vi "Sentivity Test.vi"() -> ()   [LabVIEW 2018]
uses:
  <vilib>/express/express analysis/Spectral/Block/exnSpectralBlock spectral measurements peak poly.vi
  <vilib>/express/express analysis/Spectral/Block/exnSpectralBlock spectral measurements peak DDT.vi
  <vilib>/express/express analysis/Spectral/XNode/ExpressSpectralMeasurementsBlockNode.xnode
panel:
  out "Avg For 5 Time":dbl
  out "Max @ Peak":dbl[](array[numeric])
  out "Max @ Peak":dbl
  out "Freq Hz":dbl
  in  "Test Senitivity Here":dbl=131.0
  out "FFT 2":dynamicdata(graph)
  out "TD 2":dynamicdata(graph)
  in  "Sample to Read":i32=6400
  in  "Rate":dbl=6400.0
  out "Freq Hz":dbl
  out "Max @ Peak":dbl
  out "FFT":dynamicdata(graph)
  out "TD":dynamicdata(graph)
  in  "stop (F)":bool
  # "校正器使用 394C06\n\n輸出 1g (9.8 m/s^2)\n頻率 159.2 Hz\n\n設定 5 倍取樣量 才能抓到 0.2 Hz"
  # "Senitivity set  1 mV/g in DAQmx"
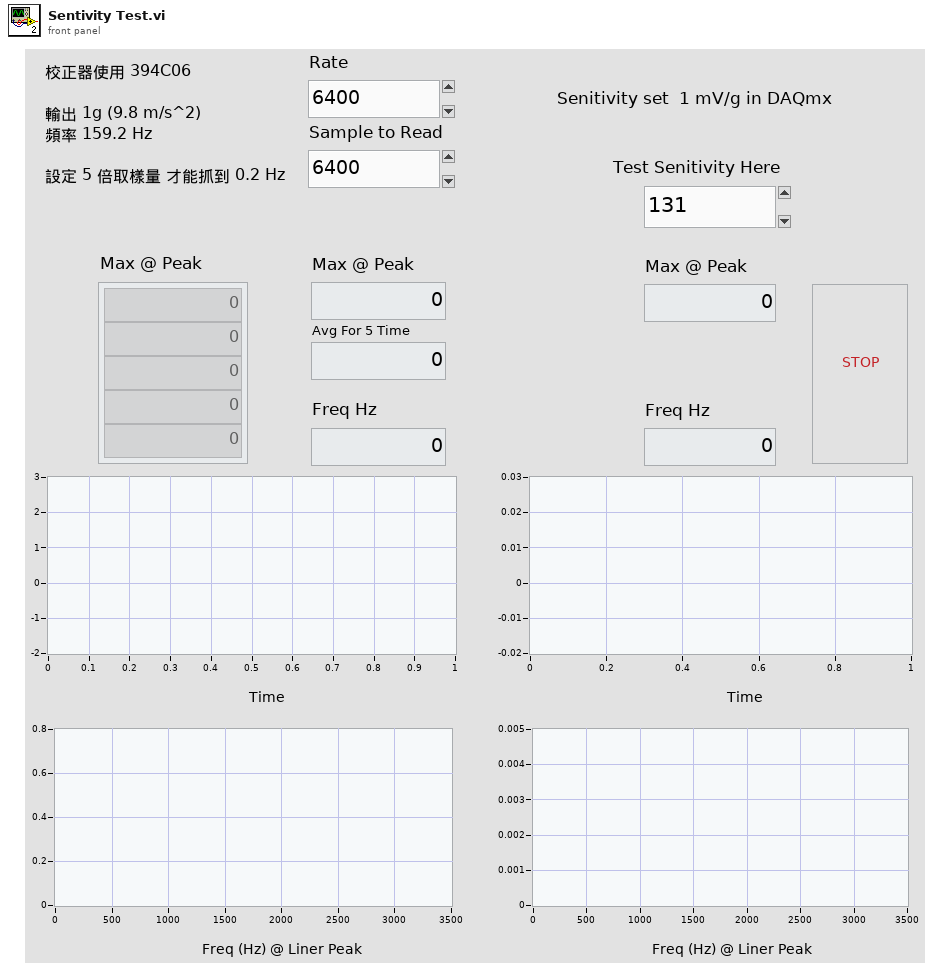
[diagram p1: front panel]
types:
  T1 = cluster{"averaging mode":u16, "weighting mode":u16, "number of averages":u32}
  T2 = cluster{"dB On (F)":bool, "unwrap phase (F)":bool, "convert to degree (F)":bool}
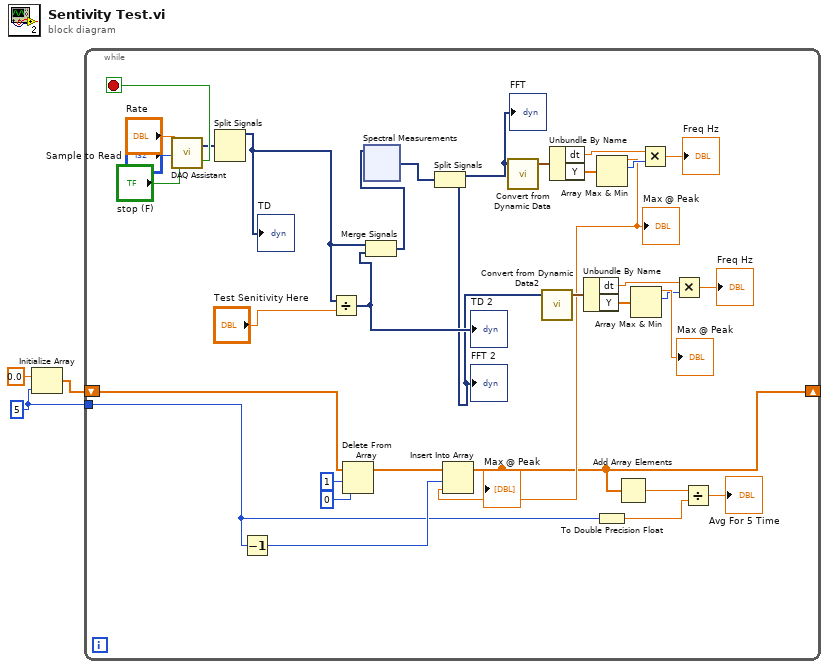
[diagram p0: block diagram]
diagram:
  w1 = 5 ("dimension size")
  n1 = Initialize Array(0.0 ("element"), w1) -> (w3:dbl[])
  n2 = while {
    shift-right: [w9] -> _
    shift-left: w3 -> [w14]
    tunnel: w1 -> [w5]
    stop <- w36 stop-if-true
    n3 = call "DAQ Assistant"("rate"="Rate", "number of samples"="Sample to Read", "stop (F)"="stop (F)") -> ("data"=w35:dynamicdata, "stopped"=w36:bool)  [unwired: 13 in, 2 out]
    n4 = Split Signals(w35) -> (w26:dynamicdata)  [unwired: 4 in, 3 out]
    "TD" <- w26
    n5 = Decrement(x=w5) -> (x-1=w6:i32)
    n6 = Divide(x=w26, y="Test Senitivity Here") -> (x/y=w22:dynamicdata)
    "TD 2" <- w22
    n7 = Delete From Array(array=w14, length=1, index=0) -> (array with subset deleted=w11:dbl[])  [unwired: 1 out]
    n8 = Merge Signals(w26, w22) -> (w25:dynamicdata)
    n9 = xnode "Spectral Measurements"("Signals"=w25) -> ("FFT - (Peak)"=w24:dynamicdata)  [unwired: 1 in, 2 out]
    n10 = Split Signals(w24) -> (w23:dynamicdata, w15:dynamicdata)  [unwired: 2 in]
    "FFT" <- w23
    "FFT 2" <- w15
    n11 = call "Convert from Dynamic Data"("Dynamic Data Type"=w23) -> ("Waveform"=w34:waveform(dbl))  [unwired: 3 in]
    n12 = call "Convert from Dynamic Data2"("Dynamic Data Type"=w15) -> ("Waveform"=w16:waveform(dbl))  [unwired: 3 in]
    n13 = Unbundle By Name(w34) -> ("dt"=w32:dbl, "Y"=w33:dbl[])
    n14 = Unbundle By Name(w16) -> ("dt"=w18:dbl, "Y"=w17:dbl[])
    n15 = Array Max & Min(array=w33) -> (max value=w10:dbl, max index (indices)=w31:i32)  [unwired: 2 out]
    "Max @ Peak" <- w10
    n16 = Insert Into Array(array=w11, index=w6, new element=w10) -> (w9:dbl[])
    "Max @ Peak" <- w9
    n17 = To Double Precision Float(number=w5) -> (double precision float=w4:dbl)
    n18 = Add Array Elements(numeric array=w9) -> (sum=w8:dbl)
    n19 = Array Max & Min(array=w17) -> (max value=→"Max @ Peak":dbl, max index (indices)=w19:i32)  [unwired: 2 out]
    n20 = Multiply(x=w32, y=w31) -> (x*y=→"Freq Hz":dbl)
    n21 = Multiply(x=w18, y=w19) -> (x*y=→"Freq Hz":dbl)
    n22 = Divide(x=w8, y=w4) -> (x/y=→"Avg For 5 Time":dbl)
  }
